vi "loadCalibration.vi"(8 "error in":errorcluster, 10 "calibration file":path, 11 "Cluster in":T1) -> (0 "error out":errorcluster, 3 "Cluster out":T1)   [LabVIEW 2020]
uses:
  controls/StateMachineVariables.ctl
  <vilib>/vision/Avi.llb/IMAQ AVI2 Refnum.ctl
  <vilib>/userDefined/High Color/IMAQdx.ctl
  <vilib>/vision/Deep Learning.llb/IMAQ DL Model Refnum.ctl
  <vilib>/vision/Image Controls.llb/IMAQ Image.ctl
  <vilib>/Utility/file.llb/Read Delimited Spreadsheet (DBL).vi
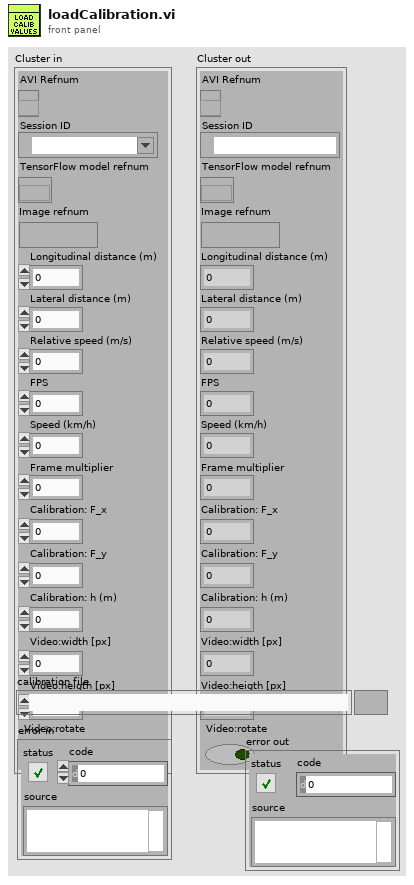
[diagram p1: front panel]
types:
  T1 = typedef "StateMachineVariables.ctl" = cluster{"AVI Refnum":T2, "Session ID":T3, "TensorFlow model refnum":T4, "Image refnum":T5, "Longitudinal distance (m)":dbl, "Lateral distance (m)":dbl, "Relative speed (m/s)":dbl, "FPS":dbl, "Speed (km/h)":dbl, "Frame multiplier":u32, "Calibration: F_x":dbl, "Calibration: F_y":dbl, "Calibration: h (m)":dbl, "Video:width [px]":i32, "Video:heigth [px]":i32, "Video:rotate":bool}
  T2 = typedef "IMAQ AVI2 Refnum.ctl" = refnum<k20>
  T3 = typedef "IMAQdx.ctl" = refnum<k21>
  T4 = typedef "IMAQ DL Model Refnum.ctl" = refnum<k20>
  T5 = typedef "IMAQ Image.ctl" = refnum<image>
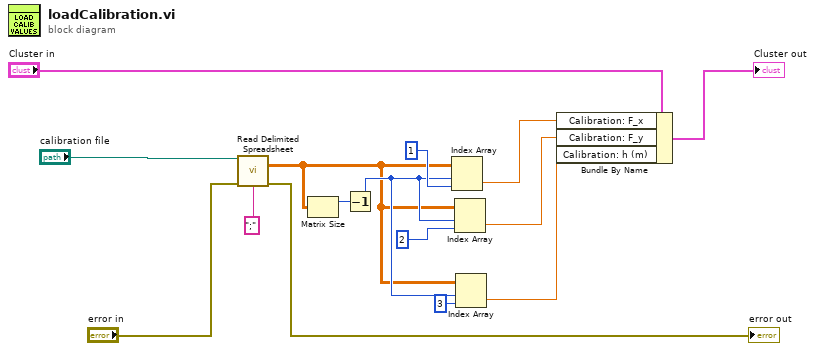
[diagram p0: block diagram]
diagram:
  n1 = call-poly <vilib>:"Read Delimited Spreadsheet.vi"("file path (dialog if empty)"="calibration file", "error in (no error)"="error in", "delimiter (\\t)"=";" ("delimiter (\\t)")) -> ("all rows"=w1:dbl[][], "error out"=→"error out":errorcluster)  [unwired: 7 in, 4 out]
  n2 = Matrix Size(0:w1) -> (1:w12:i32)  [unwired: 1 out]
  n3 = Decrement(x=w12) -> (x-1=w4:i32)
  n4 = Index Array(array=w1, index (row)=w4, index (col)=1) -> (element=w6:dbl)
  n5 = Index Array(array=w1, index (row)=w4, index (col)=2) -> (element=w5:dbl)
  n6 = Index Array(array=w1, index (row)=w4, index (col)=3) -> (element=w2:dbl)
  n7 = Bundle By Name(cluster="Cluster in", "Calibration: F_x"=w6, "Calibration: F_y"=w5, "Calibration: h (m)"=w2) -> (→"Cluster out":T1)
